vi "ma_Convert to One-sided Spectrum (real).vi"(0 "two-sided spectrum (real)":dbl[](array[numeric]) format="%0.2f") -> (1 "one-sided spectrum (real)":dbl[](array[numeric]) format="%0.2f", 2 "block size":dbl format="%0.2f")   [LabVIEW 2020, in "NI_MAPro.lvlib"]
uses:
  NI_MAPro.lvlib
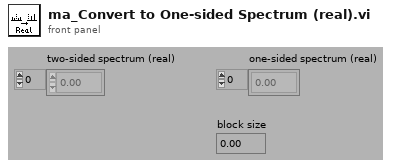
[diagram p1: front panel]
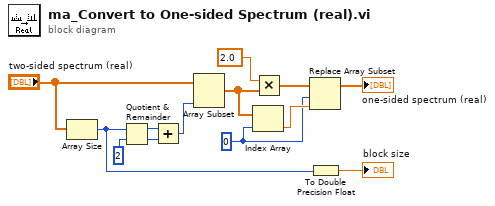
[diagram p0: block diagram]
diagram:
  w10 = 0
  n1 = Array Size(array="two-sided spectrum (real)") -> (size(s)=w4:i32)
  n2 = Quotient & Remainder(x=w4, y=2) -> (x-y*floor(x/y)=w8:i32, floor(x/y)=w7:i32)
  n3 = Add(x=w8, y=w7) -> (x+y=w6:i32)
  n4 = Array Subset(array="two-sided spectrum (real)", length=w6) -> (w3:dbl[])  [unwired: 1 in]
  n5 = Index Array(array=w3, index=w10) -> (element=w12:dbl)
  n6 = Multiply(x=2.0, y=w3) -> (x*y=w13:dbl[])
  n7 = Replace Array Subset(array=w13, new element=w12, index=w10) -> (→"one-sided spectrum (real)":dbl[])
  n8 = To Double Precision Float(number=w4) -> (double precision float=→"block size":dbl)
